vi "e-throttle.vi"(10 "potentiometer":dbl, 11 "idle":dbl) -> (3 "voltage output":dbl)   [LabVIEW 2014]
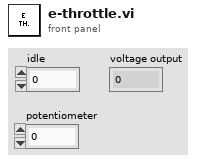
[diagram p1: front panel]
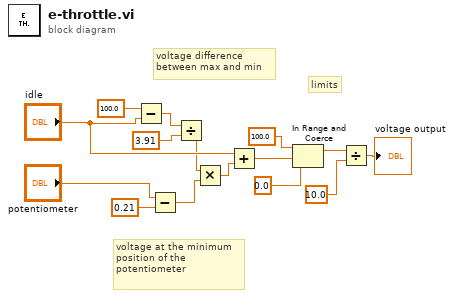
[diagram p0: block diagram]
diagram:
  # "limits"
  # "voltage at the minimum position of the potentiometer"
  # "voltage difference \nbetween max and min"
  n1 = Subtract(x=100.0, y="idle") -> (x-y=w2:dbl)
  n2 = Subtract(x="potentiometer", y=0.21) -> (x-y=w5:dbl)
  n3 = Divide(x=w2, y=3.91) -> (x/y=w4:dbl)
  n4 = Multiply(x=w4, y=w5) -> (x*y=w6:dbl)
  n5 = Add(x="idle", y=w6) -> (x+y=w12:dbl)
  n6 = In Range and Coerce(upper limit=100.0, x=w12, lower limit=0.0) -> (coerced(x)=w13:dbl)  [unwired: 1 out]
  n7 = Divide(x=w13, y=10.0) -> (x/y=→"voltage output":dbl)
